vi "_Get Named Range.vi"(7 "Sheet Name":string, 8 "error in":errorcluster, 10 "Range Identifier":string, 11 "SpreadsheetDoc in":refnum<k24>) -> (0 "error out":errorcluster, 1 "Range":string, 2 "DefinedName":refnum<k24>, 3 "SpreadsheetDoc out":refnum<k24>, 5 "Sheet Name":string)   [LabVIEW 2021, in "Open Xml.lvlib"]
uses:
  Open Xml.lvlib
  D:/git/Open-Xml-LabVIEW/dll/DocumentFormat.OpenXml.dll
  dll/DocumentFormat.OpenXml.dll
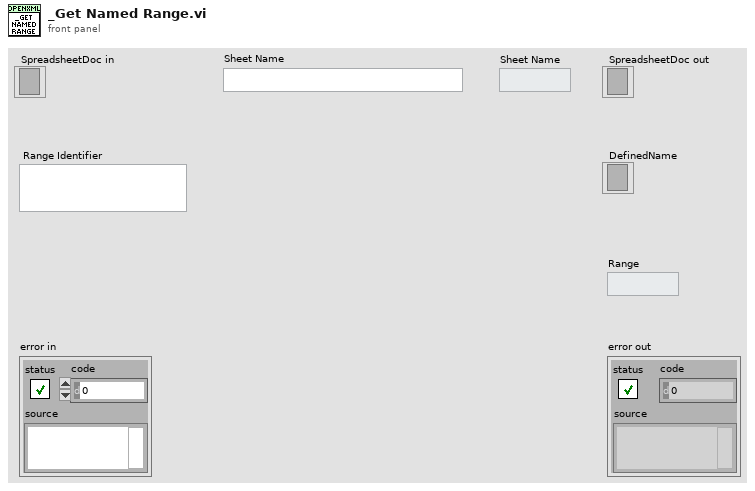
[diagram p1: front panel]
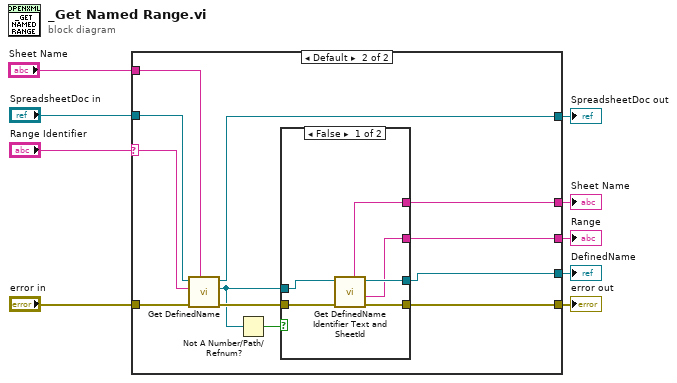
[diagram p0: block diagram]
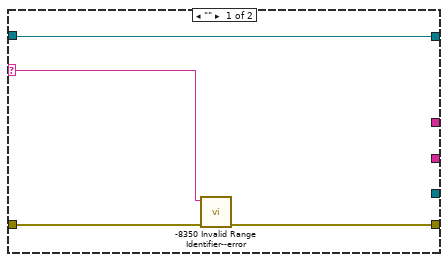
[diagram p2: hidden frame]
diagram:
  n1 = case shown="Default" "Range Identifier" {
    selector: "Range Identifier" -> [w11 w23]
    tunnel: "error in" -> [w13 w25]
    tunnel: [w12 w16] -> w8
    tunnel: "SpreadsheetDoc in" -> [w10 w19]
    tunnel: [w10 w18] -> w6
    tunnel: "Sheet Name" -> [_ w24]
    tunnel: [_ w17] -> w3
    tunnel: [_ w15] -> w2
    tunnel: [_ w14] -> w1
    frame "" {
      n2 = call "-8350 Invalid Range Identifier--error.vi"("error in"=w13, "Argument"=w11) -> ("error out"=w12:errorcluster)  [unwired: 9 in]
    }
    frame Default {
      n3 = call "Get DefinedName.vi"("Sheet Name"=w24, "error in"=w25, "Range Identifier"=w23, "SpreadsheetDoc in"=w19) -> ("error out"=w22:errorcluster, "DefinedName"=w20:refnum<k24>, "SpreadsheetDoc out"=w18:refnum<k24>)  [unwired: 4 in, 1 out]
      n4 = Not A Number/Path/Refnum?(number/path/refnum=w20) -> (NaN/Path/Refnum?=w21:bool)
      n5 = case shown="False" w21 {
        tunnel: [w31 w32] -> w14
        tunnel: w22 -> [w29 w33]
        tunnel: w20 -> [w30 w32]
        tunnel: [w28 w33] -> w16
        tunnel: [w27 _] -> w17
        tunnel: [w26 _] -> w15
        frame False {
          n6 = call "Get DefinedName Identifier Text and SheetId.vi"("error in"=w29, "DefinedName in"=w30) -> ("error out"=w28:errorcluster, "Range"=w26:string, "DefinedName out"=w31:refnum<k24>, "Sheet Name"=w27:string)  [unwired: 5 in, 1 out]
        }
        frame True {
        }
      }
    }
  }
  "error out" <- w8
  "SpreadsheetDoc out" <- w6
  "Sheet Name" <- w3
  "Range" <- w2
  "DefinedName" <- w1
